vi "TestSerpoint.vi"() -> ()   [LabVIEW 2022 SP3]
panel:
  out "Waveform Chart":waveform(dbl)(graph)
  in  "IC(BI3)":bool
  in  "ULL(AI4)":dbl
  in  "SetP Grad":dbl
  in  "ILL(AI3)":dbl
  in  "Igrd(AI1)":dbl
  in  "I-(BI1)":bool
  in  "I+(BI2)":bool
  in  "IAd(AI2)":dbl
  in  "Input":dbl
  in  "stop":bool
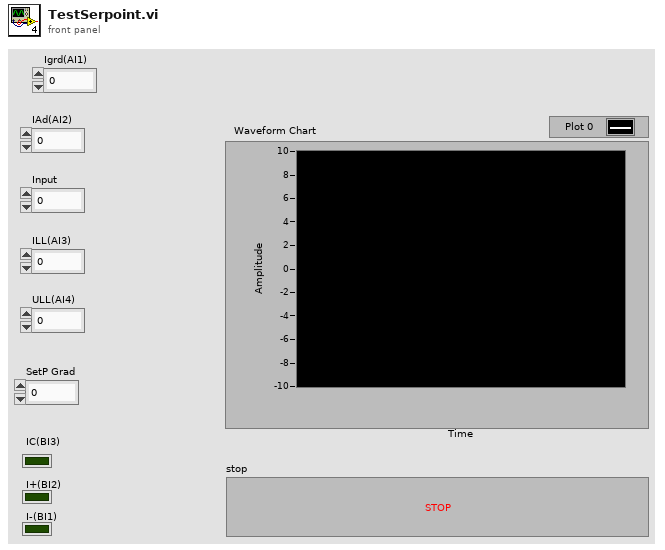
[diagram p1: front panel]
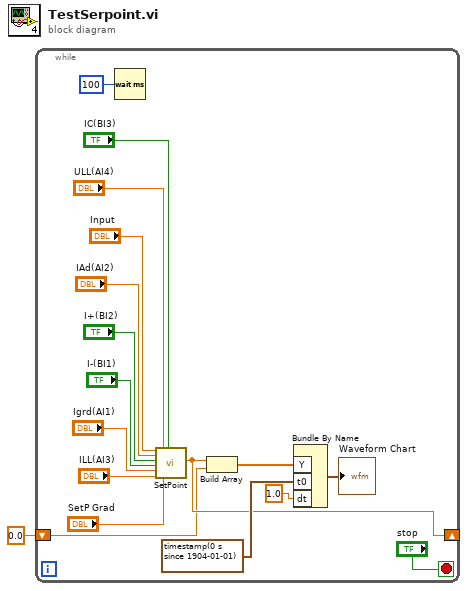
[diagram p0: block diagram]
diagram:
  n1 = while {
    shift-right: [w6] -> _
    shift-left: 0.0 ("Output (AO1)") -> [w2]
    stop <- "stop" stop-if-true
    n2 = Wait (ms)(milliseconds to wait=u32 100) -> ()  [unwired: 1 out]
    n3 = call "SetPoint.vi"("Input"="Input", "IAd(AI2)"="IAd(AI2)", "I+(BI2)"="I+(BI2)", "I-(BI1)"="I-(BI1)", "Igrd(AI1)"="Igrd(AI1)", "ILL(AI3)"="ILL(AI3)", "ULL(AI4)"="ULL(AI4)", "SetP Grad"="SetP Grad", "IC(BI3)"="IC(BI3)") -> ("Output (AO1)"=w6:dbl)  [unwired: 10 in]
    n4 = Build Array(w6, w2) -> (w5:dbl[])
    n5 = Bundle By Name("Y"=w5, "t0"=timestamp(0 s since 1904-01-01), "dt"=1.0) -> (→"Waveform Chart":waveform(dbl))  [unwired: 1 in]
  }
